vi "Send Launch Nested Actors Selector.vi"(7 "Message Priority (Normal)":T1=enum."Normal", 8 "error in (no error)":errorcluster, 10 "CTRL":refnum<vi>, 11 "Message Enqueuer":refnum<class "Message Enqueuer.lvclass">) -> (0 "error out":errorcluster, 3 "Message Enqueuer out":refnum<class "Message Enqueuer.lvclass">)   [LabVIEW 2023, in "GUI.lvlib" / "Main.lvlib" / "Launch Nested Actors Selector Msg.lvclass"]
doc: "This VI sends the message to an actor."
uses:
  Launch Nested Actors Selector Msg.lvclass
  Launch Nested Actors Selector Msg.lvclass/Launch Nested Actors Selector Msg.ctl
  <vilib>/ActorFramework/Message Enqueuer/Message Enqueuer.lvclass
  C:/Program Files/National Instruments/LabVIEW 2023/vi.lib/ActorFramework/Message/Message.lvclass
  D:/eDCU LTT/VT LTT Project/Source Code/GUI/Actor/Main/Main Messages/Launch Nested Actors Selector Msg/Launch Nested Actors Selector Msg.lvclass
  <vilib>/ActorFramework/Message Enqueuer/Message Priority.ctl
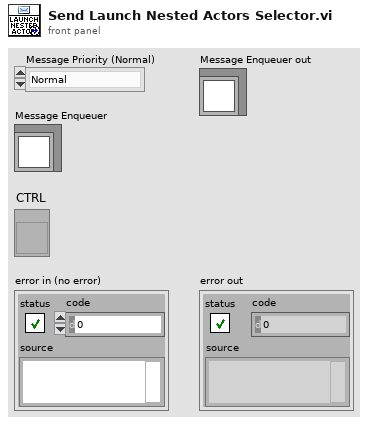
[diagram p1: front panel]
types:
  T1 = typedef "Actor Framework.lvlib/Message Enqueuer.lvclass/Message Priority.ctl" = enum16{"Low", "Normal", "High"}
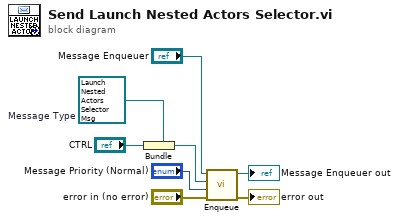
[diagram p0: block diagram]
diagram:
  w5 = refnum<class "Launch Nested Actors Selector Msg.lvclass"> refnum  # Message Type
  n1 = Bundle(cluster=w5, "CTRL") -> (w4:refnum<class "Launch Nested Actors Selector Msg.lvclass">)
  n2 = call <vilib>:"Enqueue.vi"("error in (no error)"="error in (no error)", "Message Priority (Normal)"="Message Priority (Normal)", "Message"=w4, "Message Enqueuer in"="Message Enqueuer") -> ("error out"=→"error out":errorcluster, "Message Enqueuer in"=→"Message Enqueuer out":refnum<class "Message Enqueuer.lvclass">)  [unwired: 6 in]
